vi "SubVI_TeleOpDrive_TeleOp.vi"(9 "DriveShifter":bool, 10 "X axis":dbl, 11 "Y axis":dbl) -> ()   [LabVIEW 2017]
doc: "This VI is called for each TeleOp packet received from the DS where the robot is not disabled. It is often used to read from the joysticks and update I/O or to update setpoints for timed control loops. It should complete and return within 20 milliseconds or it may miss DS packets."
uses:
  <vilib>/Rock Robotics/WPI/Utilities/WPI_GetSetVariantRefNum.vi
  <vilib>/Rock Robotics/WPI/ThirdParty/Phoenix-LabVIEW/Motor Controller/Get/CTRE_Phoenix_MotorController_GetSelectedSensorData.vi
  <vilib>/Rock Robotics/WPI/ThirdParty/Phoenix-LabVIEW/Motor Controller/Get/CTRE_Phoenix_MotorController_GetClosedLoopData.vi
  <vilib>/Rock Robotics/WPI/ThirdParty/Phoenix-LabVIEW/Motor Controller/Get/CTRE_Phoenix_MotorController_GetVoltage.vi
  <vilib>/Rock Robotics/WPI/ThirdParty/Phoenix-LabVIEW/Motor Controller/Get/CTRE_Phoenix_MotorController_GetOutputCurrent_Enhanced.vi
panel:
  out "Velocity (Raw Sensor Units per 100 ms) 6":i32
  out "Position (inches) 6":i32
  out "Percent Output 4":dbl
  out "Velocity  5":i32
  out "Position  5":i32
  out "Percent Output 3":dbl
  out "Output Current 3":dbl
  out "Closed-loop Error 4":i32
  out "Output Current 4":dbl
  out "Closed-loop Error 3":i32
  out "Position (inches) 5":i32
  out "Position (Raw Sensor Units) 6":i32
  in  "Y Multiply Spd":dbl=450.0 format="%#_13g"
  out "Y Input":dbl
  in  "DriveShiftLow":bool
  in  "X and Y values In":bool=TRUE
  in  "X axis value":dbl
  in  "Y axis value":dbl
  out "encoder position":i32(graph)
  out "X and Y":T1(graph)
  out "joystick X":dbl
  out "joystick Y":dbl
  out "closed loop error":T2(graph)
  out "voltage vs current left":T1(graph)
  out "voltage vs current right":T1(graph)
  out "Speed Closed Loop Plots":T3(graph)
  # "front panel"
  # "joystick"
  # "what we want"
  # "actual"
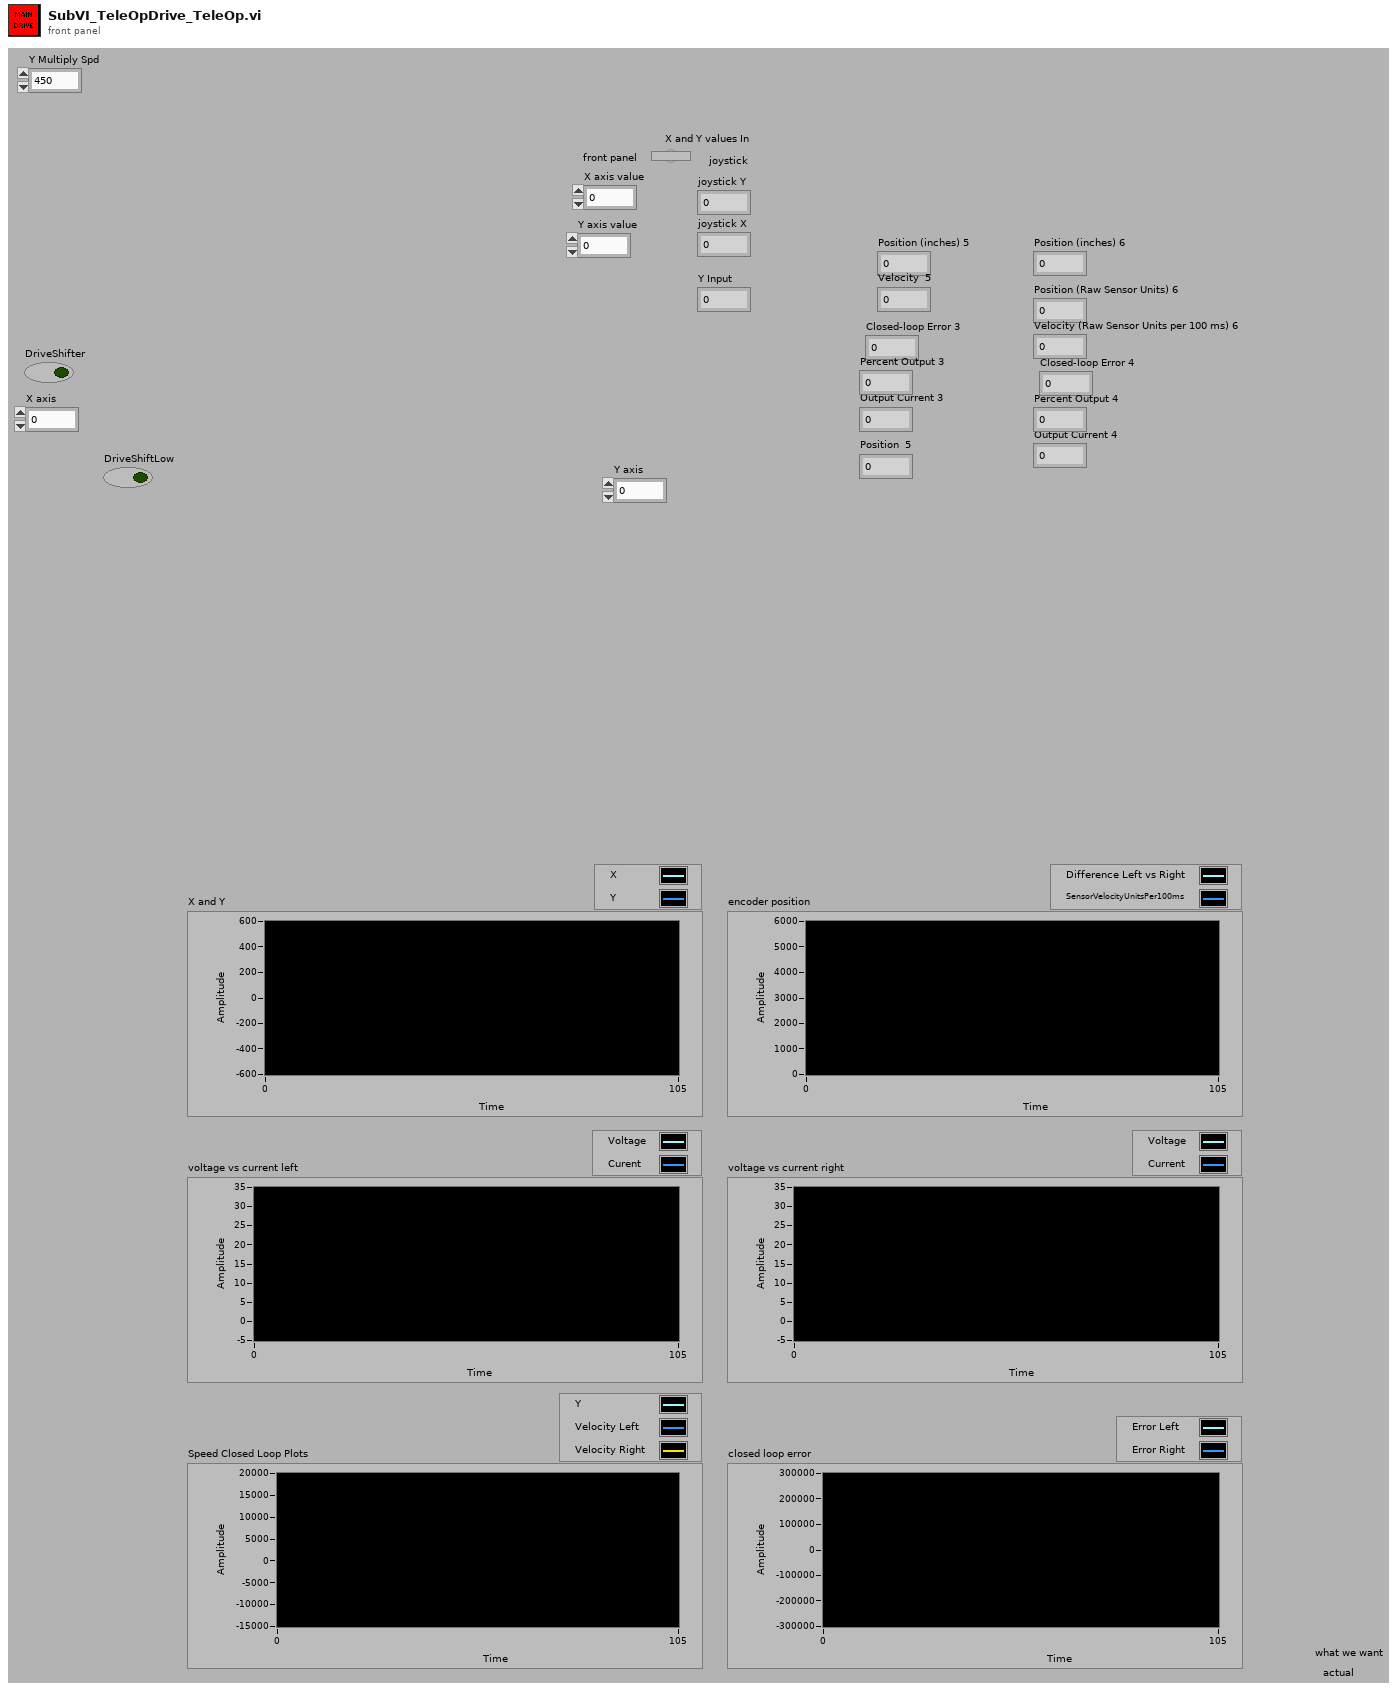
[diagram p1: front panel]
types:
  T1 = cluster{"Percent Output":dbl, "Output Current":dbl}
  T2 = cluster{"Closed-loop Error":i32, "Closed-loop Error":i32}
  T3 = cluster{dbl, "Velocity (Raw Sensor Units per 100 ms)":i32, "Velocity (Raw Sensor Units per 100 ms)":i32}
  T4 = typedef "WPI_MotorControlDeviceRef.ctl" = cluster{"DeviceStatus":errorcluster, "Type":T5, "PWM":cluster{"PWM Channel":T6, "DeadBand":T7}, "CAN":cluster{"Device Number":u8, "SetOutput VI Ref":variant, "GetOutput VI Ref":variant, "Enable VI Ref":variant, "Disable VI Ref":variant, "Data":variant}, "Invert":bool, "DIO PWM":cluster{"PWM \"Enable\" Channel":T6, "DIOChannel":T8, "PWM Rate":dbl}}
  T5 = typedef "WPI_MotorControlType.ctl" = enum16{"PWM", "CAN", "DIO PWM"}
  T6 = typedef "FPGA_DIOPWMChannel.ctl" = enum8{"PWM 0", "PWM 1", "PWM 2", "PWM 3", "PWM 4", "PWM 5", "PWM 6", "PWM 7", "PWM 8", "PWM 9", "PWM MXP 0", "PWM MXP 1", "PWM MXP 2", "PWM MXP 3", "PWM MXP 4", "PWM MXP 5", "PWM MXP 6", "PWM MXP 7", "PWM MXP 8", "PWM MXP 9", "Invalid"}
  T7 = typedef "WPI_PWMDeadband.ctl" = cluster{"Name":string, "maxPositivePwm":i32, "minPositivePwm":i32, "centerPwm":i32, "maxNegativePwm":i32, "minNegativePwm":i32, "angularRange":u16}
  T8 = typedef "FPGA_DIOChannel.ctl" = enum8{"DIO 0", "DIO 1", "DIO 2", "DIO 3", "DIO 4", "DIO 5", "DIO 6", "DIO 7", "DIO 8", "DIO 9", "DIO MXP 0", "DIO MXP 1", "DIO MXP 2", "DIO MXP 3", "DIO MXP 4", "DIO MXP 5", "DIO MXP 6", "DIO MXP 7", "DIO MXP 8", "DIO MXP 9", "DIO MXP 10", "DIO MXP 11", "DIO MXP 12", "DIO MXP 13", "DIO MXP 14", "DIO MXP 15", "SPI Port CS1", "SPI Port CS2", "SPI Port CS3", "SPI Port MISO", "SPI Port MOSI", "Invalid"}
  T9 = typedef "WPI_RobotDriveDevRef.ctl" = cluster{"DevStatus":errorcluster, "Motors[]":T4[], "Square Inputs":bool, "Max Output":dbl}
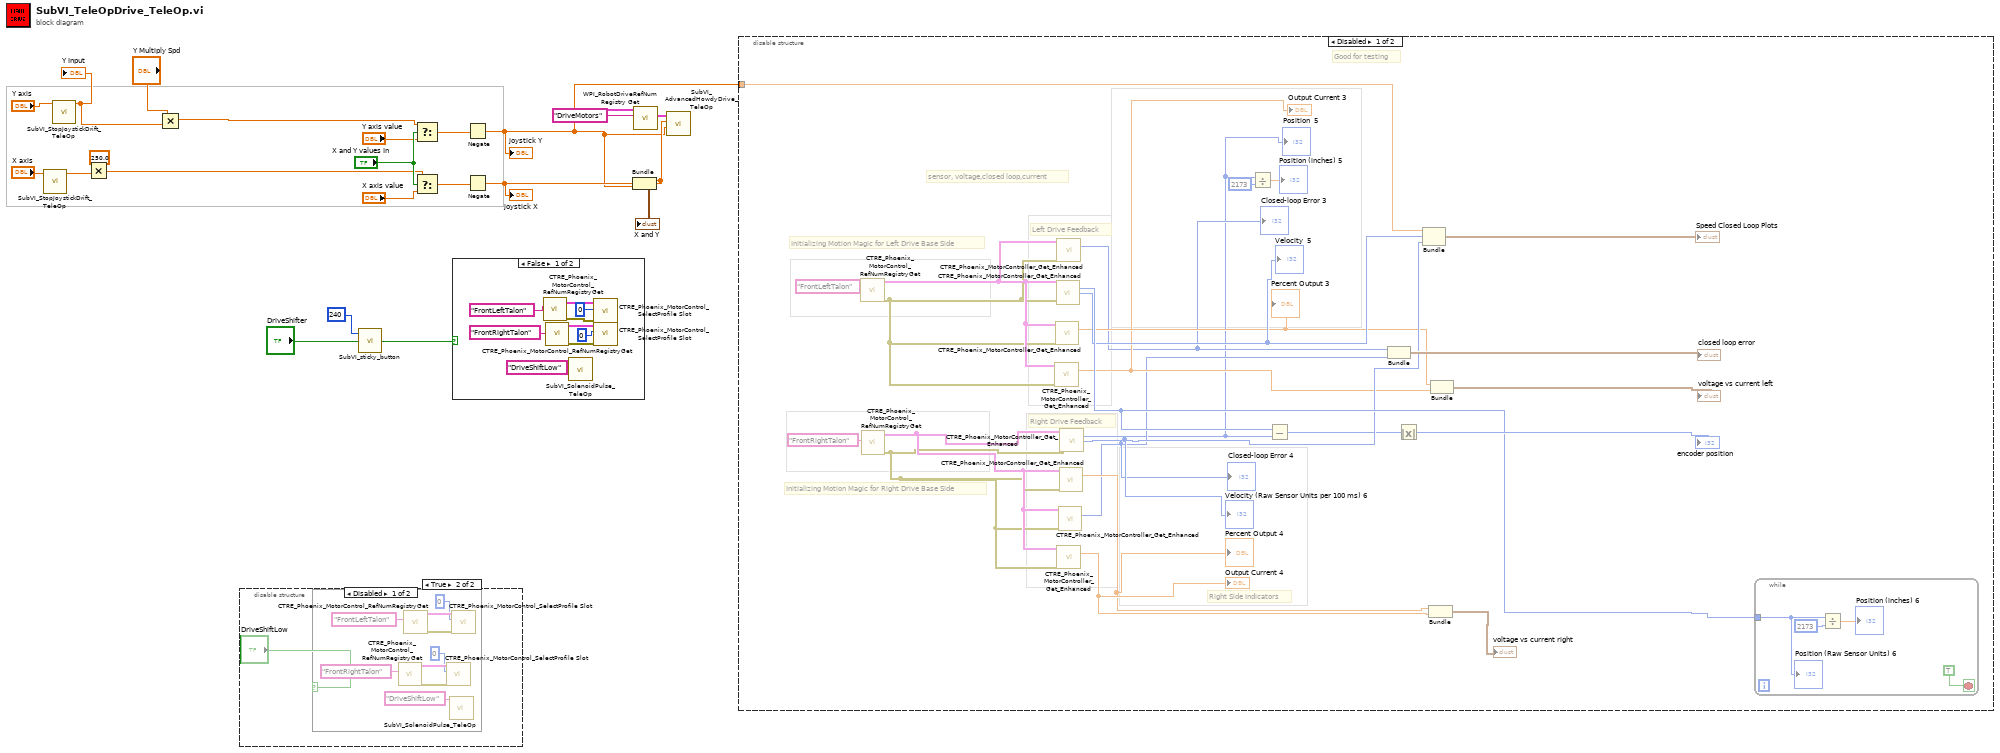
[diagram p0: block diagram]
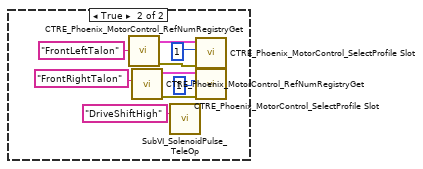
[diagram p5: hidden frame]
diagram:
  n1 = call "SubVI_StopJoystickDrift_TeleOp.vi"("upper limit in"="X axis") -> ("upper limit out"=w8:dbl)  [unwired: 10 in]
  n2 = call "SubVI_StopJoystickDrift_TeleOp.vi"("upper limit in"="Y axis") -> ("upper limit out"=w5:dbl)  [unwired: 10 in]
  "Y Input" <- w5
  n3 = Multiply(x=250.0, y=w8) -> (x*y=w6:dbl)
  n4 = Multiply(x="Y Multiply Spd", y=w5) -> (x*y=w7:dbl)
  n5 = disable-structure shown="Disabled" {
    frame Disabled {
      n6 = case shown="True" "DriveShiftLow" {
        frame False {
        }
        frame True {
          n7 = call <vilib>:"CTRE_Phoenix_MotorControl_RefNumRegistryGet.vi"("refnum name"="FrontRightTalon") -> ("error out"=w24:errorcluster, "PhoenixMotorControlDevRef"=w30:T4)  [unwired: 9 in]
          n8 = call <vilib>:"CTRE_Phoenix_MotorControl_RefNumRegistryGet.vi"("refnum name"="FrontLeftTalon") -> ("error out"=w23:errorcluster, "PhoenixMotorControlDevRef"=w29:T4)  [unwired: 9 in]
          n9 = call <vilib>:"CTRE_Phoenix_MotorControl_SelectProfile Slot.vi"("error in (no error)"=w24, "slotIdx"=0, "PhoenixMotorControlDevRef"=w30) -> ()  [unwired: 7 in, 2 out]
          n10 = call "SubVI_SolenoidPulse_TeleOp.vi"("Solenoid"="DriveShiftLow") -> ()  [unwired: 10 in, 1 out]
          n11 = call <vilib>:"CTRE_Phoenix_MotorControl_SelectProfile Slot.vi"("error in (no error)"=w23, "slotIdx"=0, "PhoenixMotorControlDevRef"=w29) -> ()  [unwired: 7 in, 2 out]
        }
      }
    }
    frame Enabled {
    }
  }
  n12 = call "SubVI_sticky_button.vi"("Speedy Input"="DriveShifter", "Number of milliseconds to wait.\n~20ms precision."=240) -> ("Sticky Output"=w3:bool)  [unwired: 1 in]
  n13 = Select(t=w7, s="X and Y values In", f="Y axis value") -> (s? t:f=w15:dbl)
  n14 = Select(t=w6, s="X and Y values In", f="X axis value") -> (s? t:f=w16:dbl)
  n15 = case shown="False" w3 {
    frame False {
      n16 = call <vilib>:"CTRE_Phoenix_MotorControl_RefNumRegistryGet.vi"("refnum name"="FrontLeftTalon") -> ("error out"=w38:errorcluster, "PhoenixMotorControlDevRef"=w32:T4)  [unwired: 9 in]
      n17 = call <vilib>:"CTRE_Phoenix_MotorControl_RefNumRegistryGet.vi"("refnum name"="FrontRightTalon") -> ("error out"=w39:errorcluster, "PhoenixMotorControlDevRef"=w40:T4)  [unwired: 9 in]
      n18 = call "SubVI_SolenoidPulse_TeleOp.vi"("Solenoid"="DriveShiftLow") -> ()  [unwired: 10 in, 1 out]
      n19 = call <vilib>:"CTRE_Phoenix_MotorControl_SelectProfile Slot.vi"("error in (no error)"=w38, "slotIdx"=0, "PhoenixMotorControlDevRef"=w32) -> ()  [unwired: 7 in, 2 out]
      n20 = call <vilib>:"CTRE_Phoenix_MotorControl_SelectProfile Slot.vi"("error in (no error)"=w39, "slotIdx"=0, "PhoenixMotorControlDevRef"=w40) -> ()  [unwired: 7 in, 2 out]
    }
    frame True {
      n21 = call <vilib>:"CTRE_Phoenix_MotorControl_RefNumRegistryGet.vi"("refnum name"="FrontLeftTalon") -> ("error out"=w46:errorcluster, "PhoenixMotorControlDevRef"=w43:T4)  [unwired: 9 in]
      n22 = call <vilib>:"CTRE_Phoenix_MotorControl_RefNumRegistryGet.vi"("refnum name"="FrontRightTalon") -> ("error out"=w42:errorcluster, "PhoenixMotorControlDevRef"=w49:T4)  [unwired: 9 in]
      n23 = call "SubVI_SolenoidPulse_TeleOp.vi"("Solenoid"="DriveShiftHigh") -> ()  [unwired: 10 in, 1 out]
      n24 = call <vilib>:"CTRE_Phoenix_MotorControl_SelectProfile Slot.vi"("error in (no error)"=w46, "slotIdx"=1, "PhoenixMotorControlDevRef"=w43) -> ()  [unwired: 7 in, 2 out]
      n25 = call <vilib>:"CTRE_Phoenix_MotorControl_SelectProfile Slot.vi"("error in (no error)"=w42, "slotIdx"=1, "PhoenixMotorControlDevRef"=w49) -> ()  [unwired: 7 in, 2 out]
    }
  }
  n26 = Negate(x=w15) -> (-x=w11:dbl)
  "joystick Y" <- w11
  n27 = Negate(x=w16) -> (-x=w12:dbl)
  "joystick X" <- w12
  n28 = Bundle(w12, w11) -> (→"X and Y":cluster{dbl, dbl})  [unwired: 1 in]
  n29 = call <vilib>:"WPI_RobotDriveRefNum Registry Get.vi"("refnum name"="DriveMotors") -> ("RobotDriveDevRef"=w20:T9)  [unwired: 1 in, 9 out]
  n30 = call "SubVI_AdvancedHowdyDrive_TeleOp.vi"("Y axis value"=w11, "X axis value"=w12, "RobotDriveDevRef"=w20) -> ()  [unwired: 7 in, 2 out]
  n31 = disable-structure shown="Disabled" {
    disable-tunnel: w11 -> [w69 _]
    frame Disabled {
      # "Good for testing"
      # "Right Drive Feedback"
      # "Left Drive Feedback"
      # "Right Side Indicators"
      # "sensor, voltage,closed loop,current"
      # "Initializing Motion Magic for Left Drive Base Side"
      # "Initializing Motion Magic for Right Drive Base Side"
      n32 = call <vilib>:"CTRE_Phoenix_MotorControl_RefNumRegistryGet.vi"("refnum name"="FrontLeftTalon") -> ("error out"=w51:errorcluster, "PhoenixMotorControlDevRef"=w53:T4)  [unwired: 9 in]
      n33 = call <vilib>:"CTRE_Phoenix_MotorControl_RefNumRegistryGet.vi"("refnum name"="FrontRightTalon") -> ("error out"=w50:errorcluster, "PhoenixMotorControlDevRef"=w52:T4)  [unwired: 9 in]
      n34 = call-poly <vilib>:"CTRE_Phoenix_MotorController_Get_Enhanced.vi"("PhoenixMotorControlDevRef"=w53, "error in"=w51) -> ("Output Current"=w60:dbl)  [unwired: 11 in, 2 out]
      "Output Current 3" <- w60
      n35 = call-poly <vilib>:"CTRE_Phoenix_MotorController_Get_Enhanced.vi"("PhoenixMotorControlDevRef"=w53, "error in"=w51) -> ("Percent Output"=w61:dbl)  [unwired: 9 in, 4 out]
      "Percent Output 3" <- w61
      n36 = call-poly <vilib>:"CTRE_Phoenix_MotorController_Get_Enhanced.vi"("PhoenixMotorControlDevRef"=w53, "error in"=w51) -> ("Position (Raw Sensor Units)"=w70:i32, "Velocity (Raw Sensor Units per 100 ms)"=w62:i32)  [unwired: 10 in, 2 out]
      "Velocity  5" <- w62
      n37 = call-poly <vilib>:"CTRE_Phoenix_MotorController_Get_Enhanced.vi"("PhoenixMotorControlDevRef"=w53, "error in"=w51) -> ("Closed-loop Error"=w59:i32)  [unwired: 8 in, 5 out]
      "Closed-loop Error 3" <- w59
      n38 = call-poly <vilib>:"CTRE_Phoenix_MotorController_Get_Enhanced.vi"("PhoenixMotorControlDevRef"=w52, "error in"=w50) -> ("Output Current"=w64:dbl)  [unwired: 11 in, 2 out]
      "Output Current 4" <- w64
      n39 = call-poly <vilib>:"CTRE_Phoenix_MotorController_Get_Enhanced.vi"("PhoenixMotorControlDevRef"=w52, "error in"=w50) -> ("Closed-loop Error"=w58:i32)  [unwired: 8 in, 5 out]
      "Closed-loop Error 4" <- w58
      n40 = call-poly <vilib>:"CTRE_Phoenix_MotorController_Get_Enhanced.vi"("PhoenixMotorControlDevRef"=w52, "error in"=w50) -> ("Percent Output"=w63:dbl)  [unwired: 9 in, 4 out]
      "Percent Output 4" <- w63
      n41 = call-poly <vilib>:"CTRE_Phoenix_MotorController_Get_Enhanced.vi"("PhoenixMotorControlDevRef"=w52, "error in"=w50) -> ("Position (Raw Sensor Units)"=w54:i32, "Velocity (Raw Sensor Units per 100 ms)"=w65:i32)  [unwired: 10 in, 2 out]
      "Position  5" <- w54
      "Velocity (Raw Sensor Units per 100 ms) 6" <- w65
      n42 = Divide(x=w54, y=2173) -> (x/y=→"Position (inches) 5":dbl)
      n43 = Subtract(x=w70, y=w54) -> (x-y=w57:i32)
      n44 = Bundle("Closed-loop Error"=w59, "Closed-loop Error"=w58) -> (→"closed loop error":T2)  [unwired: 1 in]
      n45 = Absolute Value(x=w57) -> (abs(x)=→"encoder position":i32)
      n46 = Bundle(w69, "Velocity (Raw Sensor Units per 100 ms)"=w62, "Velocity (Raw Sensor Units per 100 ms)"=w65) -> (→"Speed Closed Loop Plots":T3)  [unwired: 1 in]
      n47 = Bundle("Percent Output"=w63, "Output Current"=w64) -> (→"voltage vs current right":T1)  [unwired: 1 in]
      n48 = Bundle("Percent Output"=w61, "Output Current"=w60) -> (→"voltage vs current left":T1)  [unwired: 1 in]
      n49 = while {
        tunnel: w70 -> [w75]
        stop <- TRUE stop-if-true
        n50 = Divide(x=w75, y=2173 ("x")) -> (x/y=→"Position (inches) 6":dbl)
        "Position (Raw Sensor Units) 6" <- w75
      }
    }
    frame Enabled {
    }
  }
